vi "arrays.vi"() -> (1 "appended array 2":string[][](array[string]))   [LabVIEW 2020]
panel:
  out "Which Button?":T1(ring)=enum."Center Button"
  in  "Array":string[](array[string])
  out "Numeric":dbl
  out "appended array":dbl[][](array[numeric])
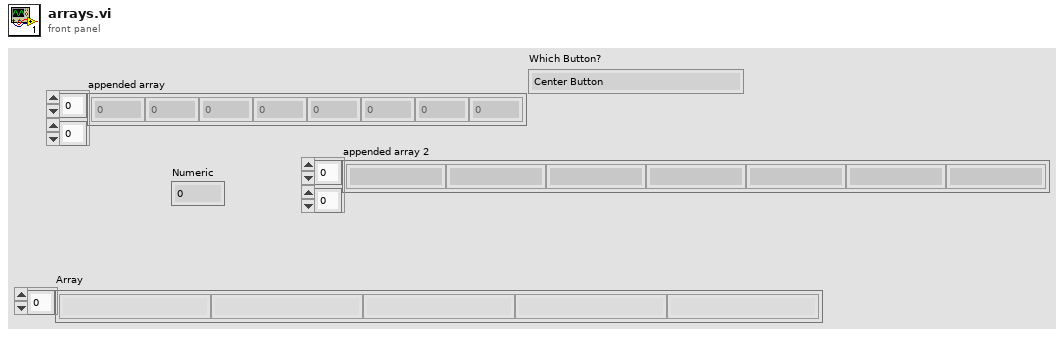
[diagram p1: front panel]
types:
  T1 = enum16{"Left Button", "Center Button", "Right Button", "Window Close"}
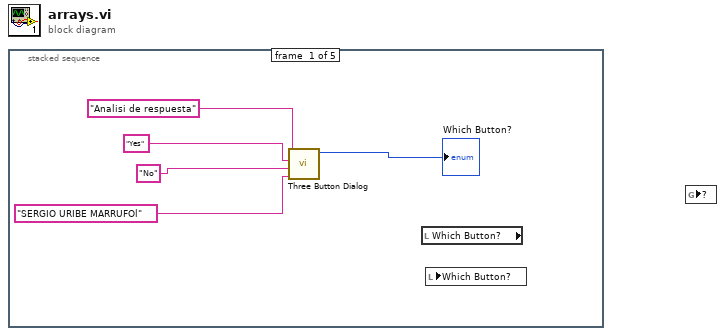
[diagram p0: block diagram]
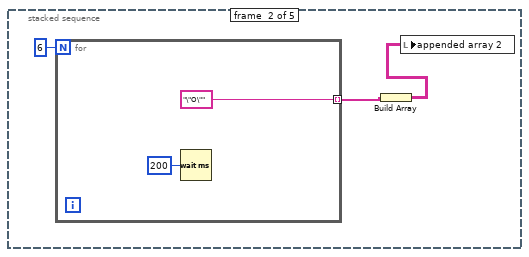
[diagram p2: hidden frame]
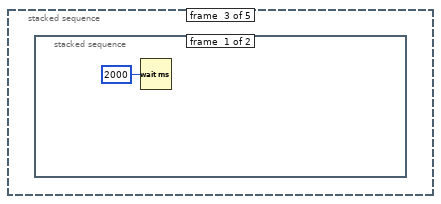
[diagram p3: hidden frame]
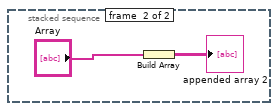
[diagram p4: hidden frame]
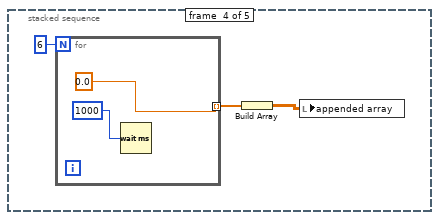
[diagram p5: hidden frame]
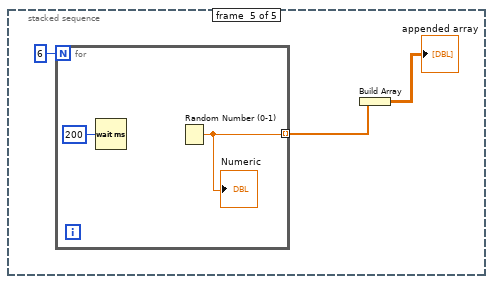
[diagram p6: hidden frame]
diagram:
  n1 = stacked-sequence {
    frame #0 {
      n2 = call <vilib>:"Three Button Dialog.vi"("Right Button Text (\"Cancel\")"="SERGIO URIBE MARRUFOl" ("Right Button Text (\"Cancel\")"), "Center Button Text (\"No\")"="No" ("Center Button Text (\"No\")"), "Left Button Text (\"Yes\")"="Yes" ("Left Button Text (\"Yes\")"), "message"="Analisi de respuesta") -> ("Which Button?"=→"Which Button?":T1)  [unwired: 7 in]
      n3 = local read "Which Button?"() -> ()  [unwired: 1 out]
      n4 = local read "Which Button?"() -> ()  [unwired: 1 in]
    }
    frame #1 {
      n5 = for {
        N: 6 -> [_]
        tunnel: ["\"O\""] -> w7 mode=indexing
        n6 = Wait (ms)(milliseconds to wait=u32 200) -> ()  [unwired: 1 out]
      }
      n7 = Build Array(w7) -> (w6:string[][])
      n8 = local write "appended array 2"(w6) -> ()
    }
    frame #2 {
      n9 = stacked-sequence {
        frame #0 {
          n10 = Wait (ms)(milliseconds to wait=u32 2000) -> ()  [unwired: 1 out]
        }
        frame #1 {
          n11 = Build Array("Array") -> (→"appended array 2":string[][])
        }
      }
    }
    frame #3 {
      n12 = for {
        N: 6 -> [_]
        tunnel: [0.0] -> w15 mode=indexing
        n13 = Wait (ms)(milliseconds to wait=u32 1000) -> ()  [unwired: 1 out]
      }
      n14 = Build Array(w15) -> (w14:dbl[][])
      n15 = local write "appended array"(w14) -> ()
    }
    frame #4 {
      n16 = for {
        N: 6 -> [_]
        tunnel: [w22] -> w20 mode=indexing
        n17 = Wait (ms)(milliseconds to wait=u32 200) -> ()  [unwired: 1 out]
        n18 = Random Number (0-1)() -> (number: 0 to 1=w22:dbl)
        "Numeric" <- w22
      }
      n19 = Build Array(w20) -> (→"appended array":dbl[][])
    }
  }
  n20 = global read "arrays.vi" item#-1() -> ()  [unwired: 1 in]
